vi "buttontoggle2.vi"(1 "Button Input":bool) -> (0 "Toggled output":bool)   [LabVIEW 2011]
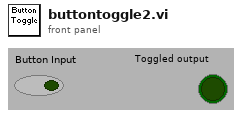
[diagram p1: front panel]
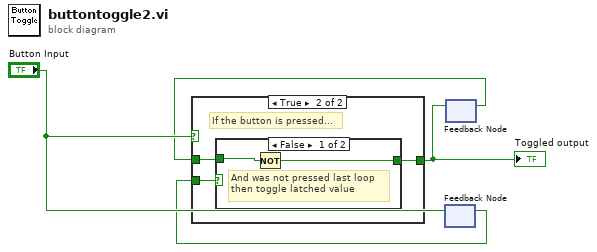
[diagram p0: block diagram]
diagram:
  n1 = feedback-in #1("Button Input") -> ()
  n2 = feedback #1() -> (w1:bool)  [unwired: 1 out]
  n3 = feedback #2() -> (w2:bool)  [unwired: 1 out]
  n4 = case shown="True" "Button Input" {
    tunnel: [w5 w8] -> w3
    tunnel: w2 -> [w5 w7]
    tunnel: w1 -> [_ w6]
    frame False {
      # "then do nothing"
      # "If button is not pressed"
    }
    frame True {
      # "If the button is pressed..."
      n5 = case shown="False" w6 {
        tunnel: [w10 w11] -> w8
        tunnel: w7 -> [w9 w11]
        frame False {
          # "And was not pressed last loop\nthen toggle latched value"
          n6 = Not(x=w9) -> (.not. x?=w10:bool)
        }
        frame True {
          # "And was pressed last loop\nthen hold current latched value"
        }
      }
    }
  }
  "Toggled output" <- w3
  n7 = feedback-in #2(w3) -> ()
